vi "Save Failure to DB.vi"(8 "error in":errorcluster, 10 "GTron DB":path=path "D:/SQL Database/Gtron Database.db", 11 "Array":string[][](array[string])) -> (0 "error out":errorcluster)   [LabVIEW 2019, in "DataLogger.lvclass"]
doc: "Save Failure Details"
uses:
  DataLogger.lvclass
  <vilib>/drjdpowell/SQLite Library/SQL Connection/Open (path).vi
  <vilib>/drjdpowell/SQLite Library/SQL Statement/SQL Statement.lvclass
  <vilib>/drjdpowell/SQLite Library/SQL Connection/Connection.lvclass
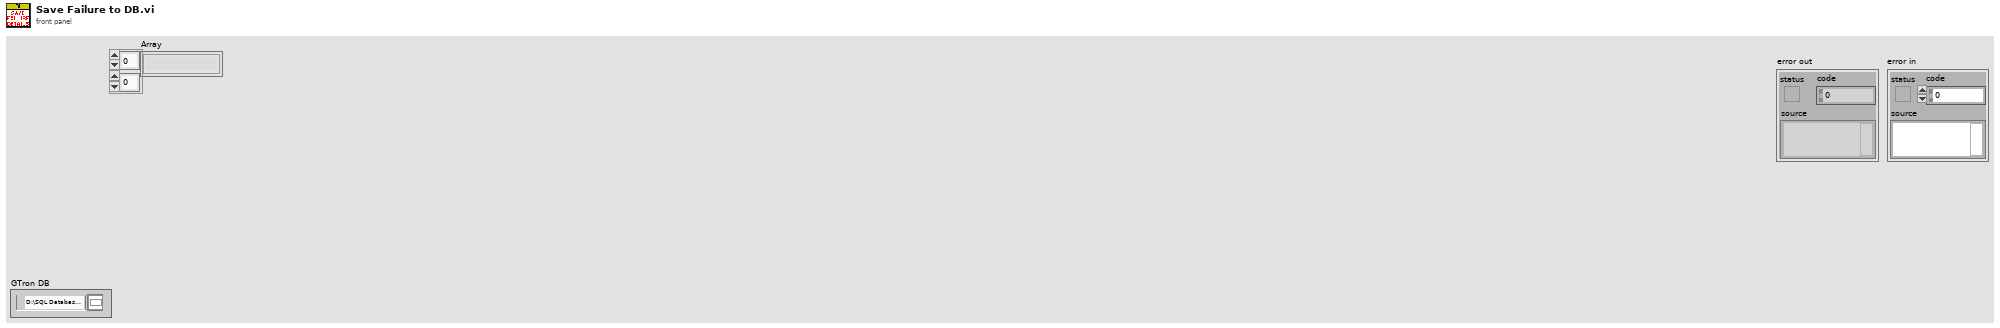
[diagram p1: front panel]
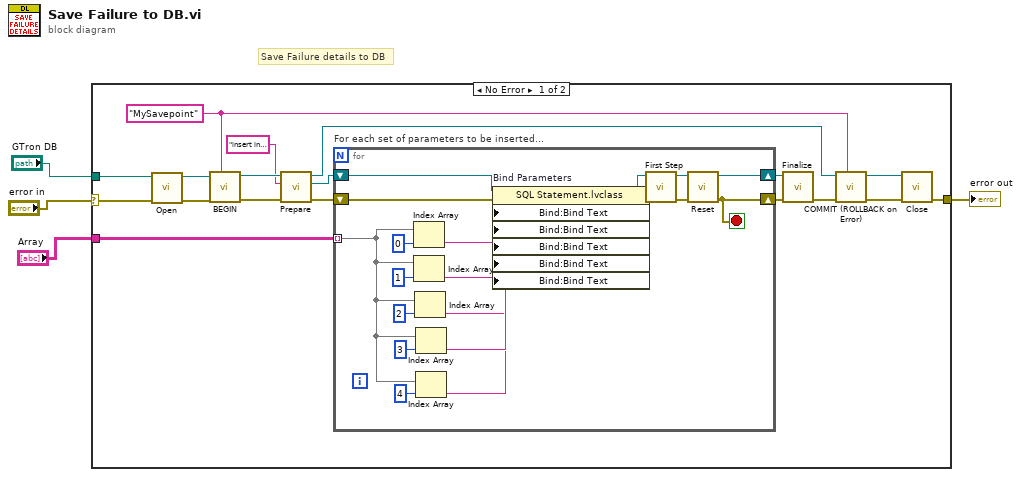
[diagram p0: block diagram]
diagram:
  # "Save Failure details to DB"
  n1 = case shown="No Error" "error in" {
    selector: "error in" -> [w6 w42]
    tunnel: "GTron DB" -> [w11 _]
    tunnel: [w10 w42] -> w3
    tunnel: "Array" -> [w5 _]
    frame No Error {
      w14 = "MySavepoint" ("Savepoint name")
      n2 = call-poly <vilib>:"Open.vi"("error in (no error)"=w6, "db file"=w11) -> ("error out"=w22:errorcluster, "SQLite Connection"=w21:refnum<class "Connection.lvclass">)  [unwired: 8 in]
      n3 = call <vilib>:"BEGIN.vi"("Savepoint name"=w14, "error in (no error)"=w22, "Connection in"=w21) -> ("error out"=w15:errorcluster, "Connection out"=w16:refnum<class "Connection.lvclass">)  [unwired: 7 in]
      n4 = call <vilib>:"Prepare.vi"("error in (no error)"=w15, "SQL"="insert into FailureDetails  VALUES (?,?,?,?,?)" ("INSERT statement"), "SQLite Connection in"=w16) -> ("error out"=w19:errorcluster, "SQL Statement"=w20:refnum<class "SQL Statement.lvclass">, "SQLite Connection"=w13:refnum<class "Connection.lvclass">)  [unwired: 4 in, 2 out]
      n5 = for "For each set of parameters to be inserted..." {
        shift-right: [w39] -> w18
        shift-left: w20 -> [w41]
        shift-right: [w38] -> w17
        shift-left: w19 -> [w40]
        tunnel: w5 -> [w24] mode=indexing
        stop <- w38 stop-if-true
        n6 = Index Array(array=w24, index=0) -> (element=w29:string)
        n7 = Index Array(array=w24, index=1) -> (element=w28:string)
        n8 = Index Array(array=w24, index=2) -> (element=w26:string)
        n9 = Index Array(array=w24, index=3) -> (element=w27:string)
        n10 = Index Array(array=w24, index=4) -> (element=w25:string)
        n11 = property on="Bind Parameters" class="SQL Statement.lvclass"(reference=w41, error in=w40, "Bind:Bind Text"=w29, "Bind:Bind Text"=w28, "Bind:Bind Text"=w26, "Bind:Bind Text"=w27, "Bind:Bind Text"=w25) -> (reference out=w37:refnum<class "SQL Statement.lvclass">, error out=w36:errorcluster)
        n12 = call <vilib>:"First Step.vi"("error in (no error)"=w36, "SQL Statement in"=w37) -> ("error out"=w35:errorcluster, "SQL Statement"=w34:refnum<class "SQL Statement.lvclass">)  [unwired: 7 in, 1 out]
        n13 = call <vilib>:"Reset.vi"("error in (no error)"=w35, "SQL Statement in"=w34) -> ("error out"=w38:errorcluster, "SQL Statement"=w39:refnum<class "SQL Statement.lvclass">)  [unwired: 8 in]
      }
      n14 = call <vilib>:"Finalize.vi"("error in (no error)"=w17, "SQL Statement in"=w18) -> ("error out"=w12:errorcluster)  [unwired: 9 in]
      n15 = call <vilib>:"COMMIT (ROLLBACK on Error).vi"("Savepoint name"=w14, "error in (no error)"=w12, "Connection in"=w13) -> ("error out"=w8:errorcluster, "Connection out"=w9:refnum<class "Connection.lvclass">)  [unwired: 7 in]
      n16 = call-dynamic "Close.vi"("error in (no error)"=w8, "SQLite Connection in"=w9) -> ("error out"=w10:errorcluster)  [unwired: 9 in]
    }
    frame Error {
    }
  }
  "error out" <- w3
